vi "Create Sig Per Frame Array.vi"(0 "Device Error":errorcluster, 11 "XNET Output Signal Names":string[](array[string])) -> (1 "Num of Sig Per Frame":i32[](array[numeric]), 2 "Number of Different Output Frames":i32, 3 "Max Number of Signals Per Frame":i32, 8 "error out":errorcluster)   [LabVIEW 2009]
uses:
  <vilib>/xnet/xnet.llb/XNET String To IO Name (Signal).vi
  Program Files/National Instruments/LabVIEW 2009/resource/objmgr/xnet.rc
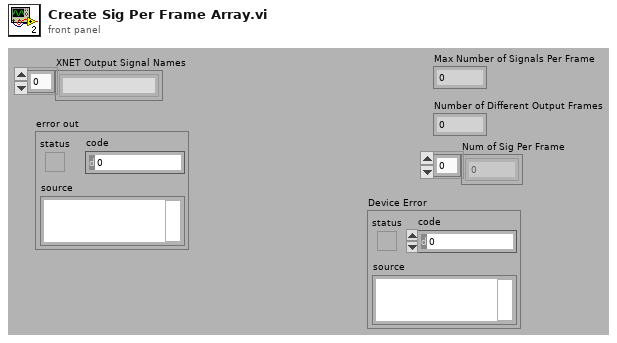
[diagram p1: front panel]
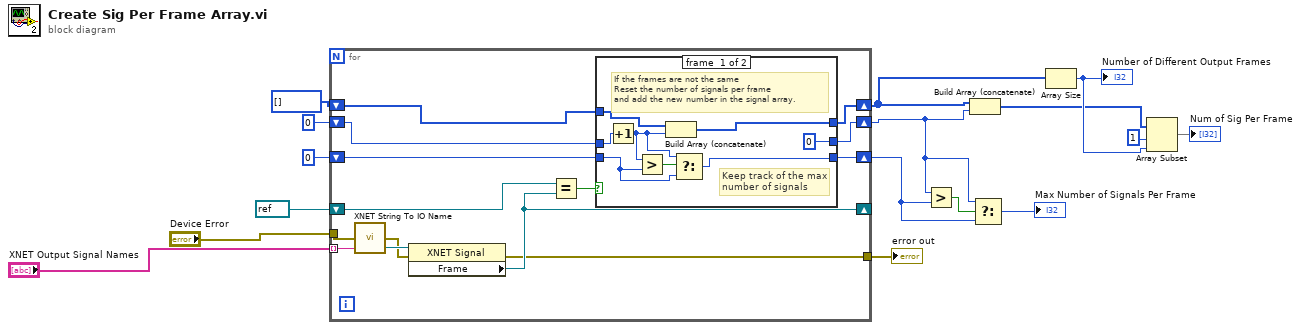
[diagram p0: block diagram]
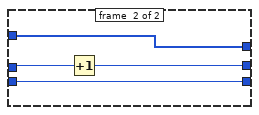
[diagram p2: hidden frame]
diagram:
  n1 = for {
    tunnel: "XNET Output Signal Names" -> [w29] mode=indexing
    shift-right: [w26] -> _
    shift-left: refnum<k21> refnum ("Frame") -> [w27]
    tunnel: "Device Error" -> [w25]
    tunnel: [w24] -> w15
    shift-right: [w19] -> w2
    shift-left: 0 -> [w22]
    shift-right: [w20] -> w3
    shift-left: i32[] [] -> [w21]
    shift-right: [w17] -> w8
    shift-left: 0 -> [w18]
    n2 = call-poly <vilib>:"XNET String To IO Name.vi"("string"=w29) -> ("XNET Signal"=w28:refnum<k21>)  [unwired: 4 in]
    n3 = property class="XNET Signal"(reference=w28, error in=w25) -> (error out=w24:errorcluster, "Frame"=w26:refnum<k21>)  [unwired: 1 out]
    n4 = Equal?(x=w27, y=w26) -> (x = y?=w23:bool)
    n5 = case shown="False" w23 {
      tunnel: [w37 w39] -> w20
      tunnel: w22 -> [w32 w41]
      tunnel: w21 -> [w30 w39]
      tunnel: [0 w40] -> w19
      tunnel: w18 -> [w34 w38]
      tunnel: [w33 w38] -> w17
      frame #0 {
        # "If the frames are not the same\nReset the number of signals per frame\nand add the new number in the signal array."
        # "Keep track of the max\nnumber of signals"
        n6 = Increment(x=w32) -> (x+1=w31:i32)
        n7 = Greater?(x=w31, y=w34) -> (0:w35:bool)
        n8 = Build Array (concatenate)(w30, w31) -> (w37:i32[])
        n9 = Select(t=w31, s=w35, f=w34) -> (s? t:f=w33:i32)
      }
      frame #1 {
        n10 = Increment(x=w41) -> (x+1=w40:i32)
      }
    }
  }
  "error out" <- w15
  n11 = Greater?(x=w2, y=w8) -> (0:w9:bool)
  n12 = Build Array (concatenate)(w3, w2) -> (w4:i32[])
  n13 = Select(t=w2, s=w9, f=w8) -> (s? t:f=→"Max Number of Signals Per Frame":i32)
  n14 = Array Size(array=w3) -> (size(s)=w5:i32)
  "Number of Different Output Frames" <- w5
  n15 = Array Subset(array=w4, index=1, length=w5) -> (→"Num of Sig Per Frame":i32[])
